vi "Module - Page Login.vi"(11 "Stop":bool) -> ()   [LabVIEW 2020]
uses:
  Control/State - eFGV.ctl
  visinergy_PRSB1-vsys-platform-6e171cc53fe6/VI/HMI/Control/State - Page Login.ctl
  <vilib>/addons/database/NI_Database_API.lvlib
  <vilib>/addons/database/Connection.llb/Conn ObjectReference.ctl
  <vilib>/addons/database/Connection.llb/DB Tools Open Connec (String).vi
  Control/Active Dir Info.ctl
panel:
  out "DB Connected":bool=TRUE
  in  "String.StationID":string
  in  "Button.Stop":bool
  in  "RSS Operation":T1(ring)
  in  "Button.Login":bool
  in  "ComboBox.Domain":string(combo) caption="Domain"
  in  "String.Password":string caption="Password"
  in  "String.Username":string caption="Username"
  in  "String.StationDescription":string
  in  "ComboBox.Station":string(combo) caption="Station"
  in  "String.PlantDescription":string
  in  "ComboBox.Plant":string(combo) caption="Plant"
  in  "Button.ConnectDB":bool
  out "2D data":string[][](array[string])
  in  "DB Connection Info":T2={"Connection"="SRTRS", "Username"="srtrsoss", "Password"="12345"}
  out "standard output":string
  out "Logon OK":bool
  out "Active Dir. Info":T3
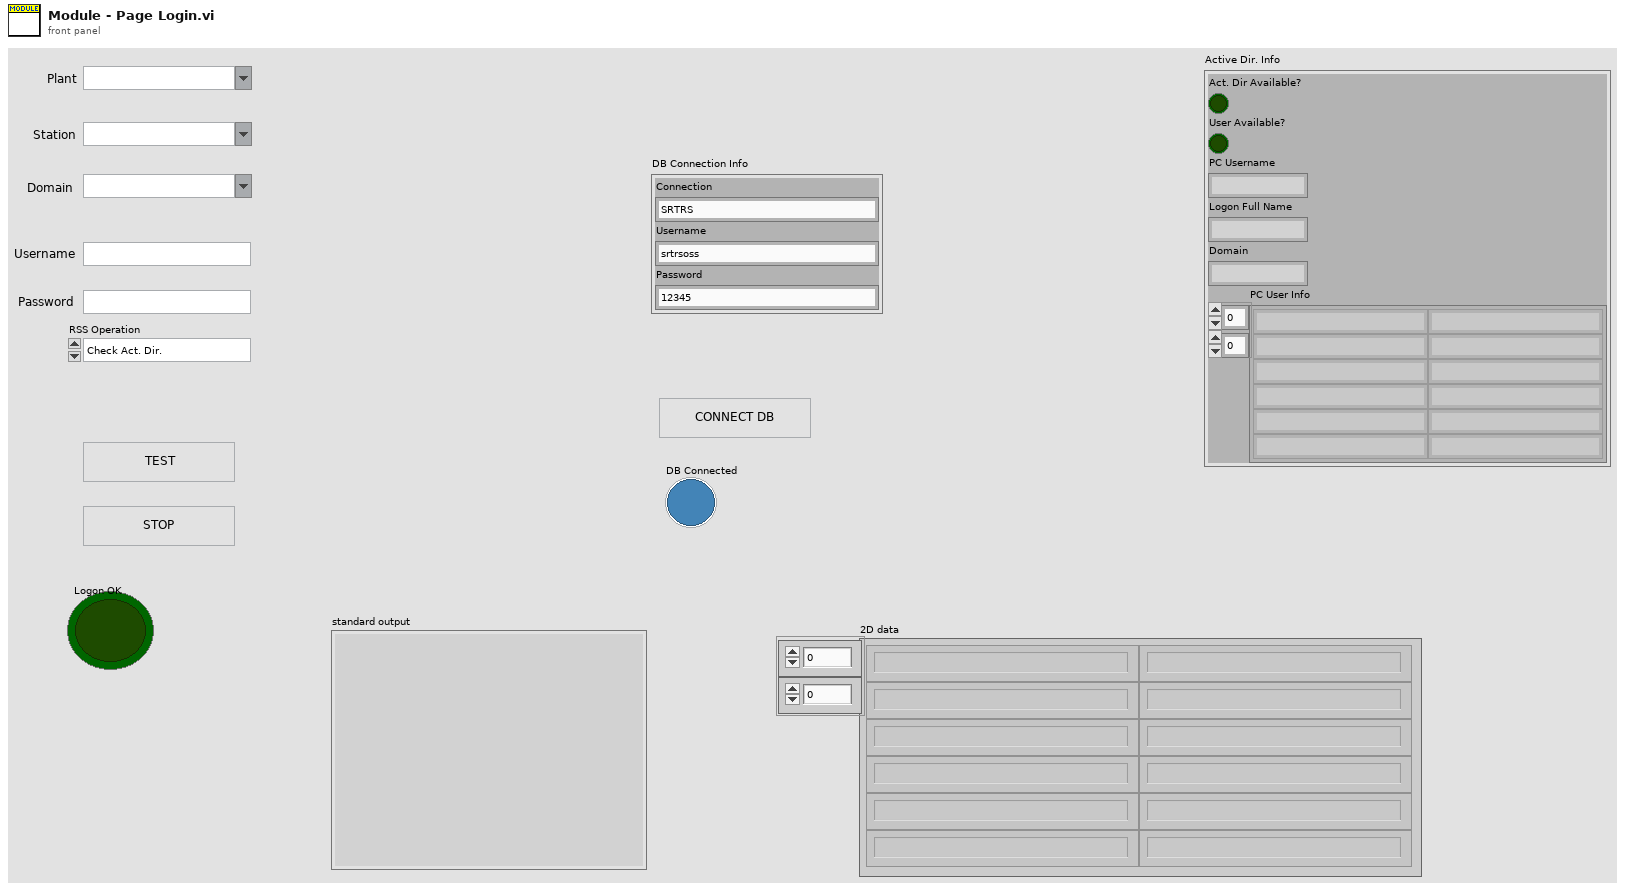
[diagram p1: front panel]
types:
  T1 = enum16{"Check Act. Dir.", "Logon", "PC User", "PC User Info", "Hostname"}
  T2 = cluster{"Connection":string, "Username":string, "Password":string}
  T3 = typedef "Active Dir Info.ctl" = cluster{"Act. Dir Available?":bool, "User Available?":bool, "PC Username":string, "Logon Full Name":string, "Domain":string, "PC User Info":string[][]}
  T4 = typedef "NI_Database_API.lvlib/Conn ObjectReference.ctl" = refnum<k1>
  T5 = cluster{"T_Out":i32, "Event Ref":refnum<event-registration>, "DB Connection Ref":T4, "2D data":string[][]}
  T6 = typedef "State - Page Login.ctl" = enum16{"Init", "Register Event", "Open DB Ref", "Get Info - Plant And Station", "Get Info - Domain", "Idle", "Login", "Close"}
  T7 = typedef "State - eFGV.ctl" = enum16{"Init", "Read", "Write", "Exit"}
  T8 = typedef "eventvkey.ctl" = enum16{"ASCII", "Enter", "Return", "Shift", "Ctrl", "Alt", "Cmd", "Opt", "Caps", "NumLock", "Clear", "Break", "Up", "Down", "Left", "Right", "Insert", "Delete", "Home", "End", "PageUp", "PageDown", "Escape", "Help", "Pause", "ScrollLock", "F1", "F2", "F3", "F4", "F5", "F6", "F7", "F8", "F9", "F10", "F11", "F12", "F13", "F14", "F15", "F16", "F17", "F18", "F19", "F20", "F21", "F22", "F23", "F24", "Play", "VolumeUp", "VolumeDown", "Mute", "Two Byte Char"}
  T9 = enum32{"invalid app kind", "Development System", "Run Time System", "Student Edition", "Embedded LabVIEW", "Evaluation", "Custom"}
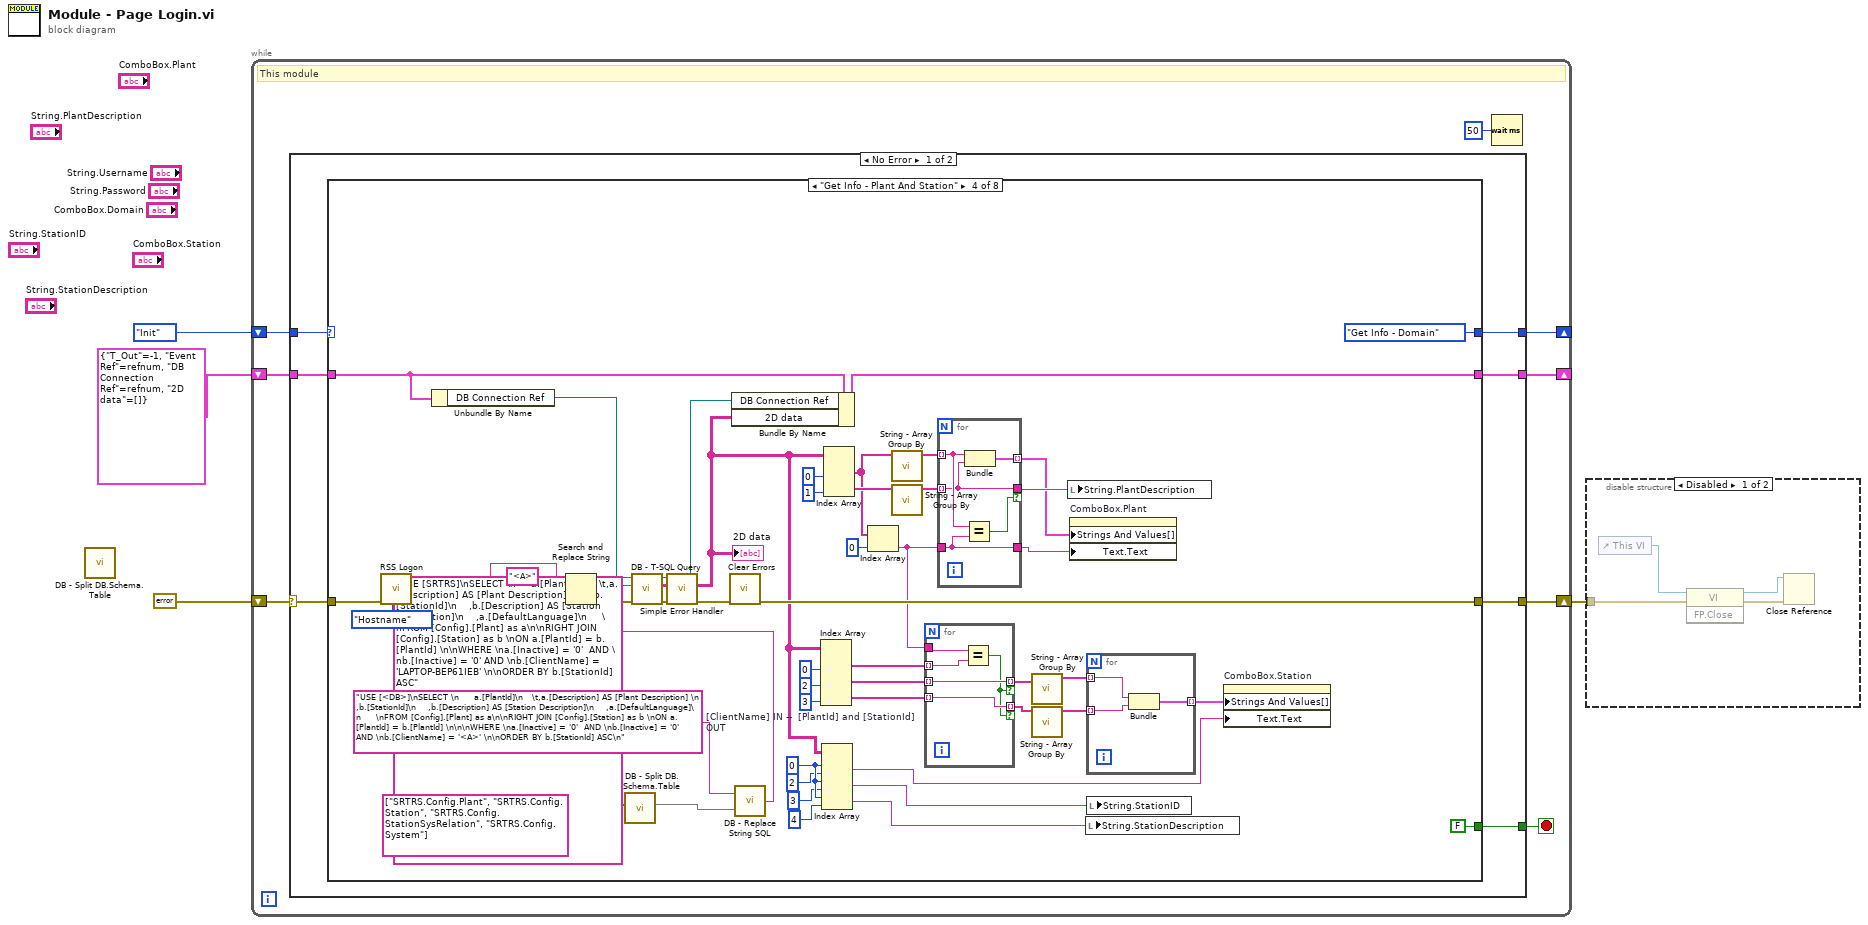
[diagram p0: block diagram]
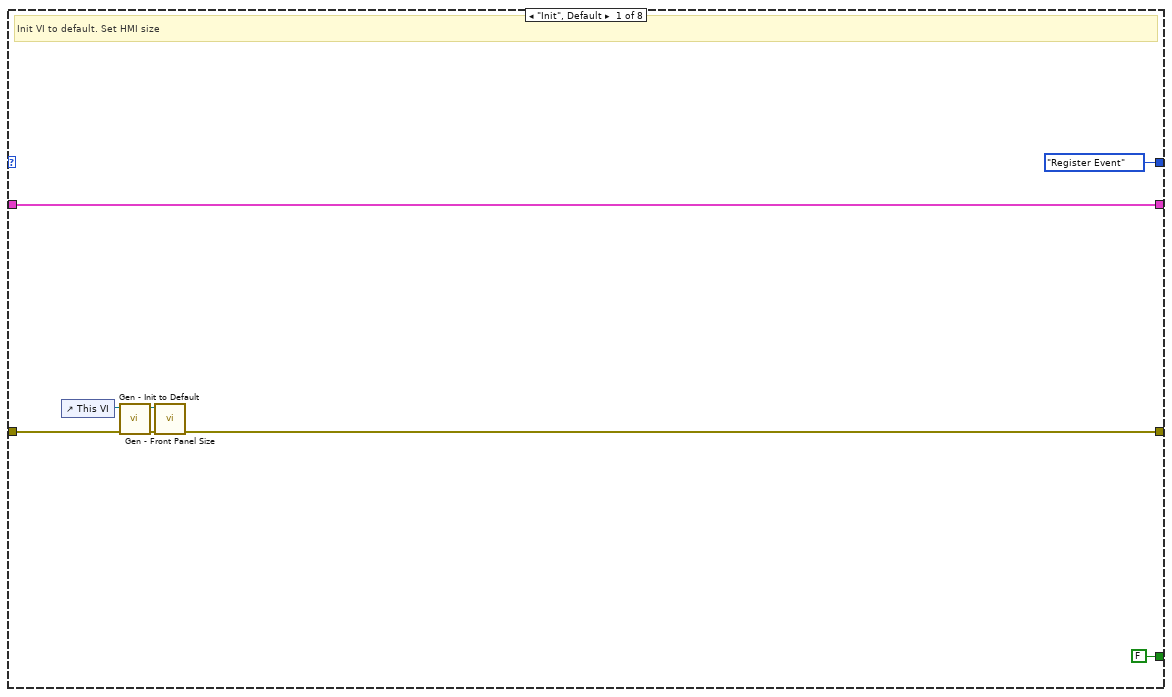
[diagram p3: hidden frame]
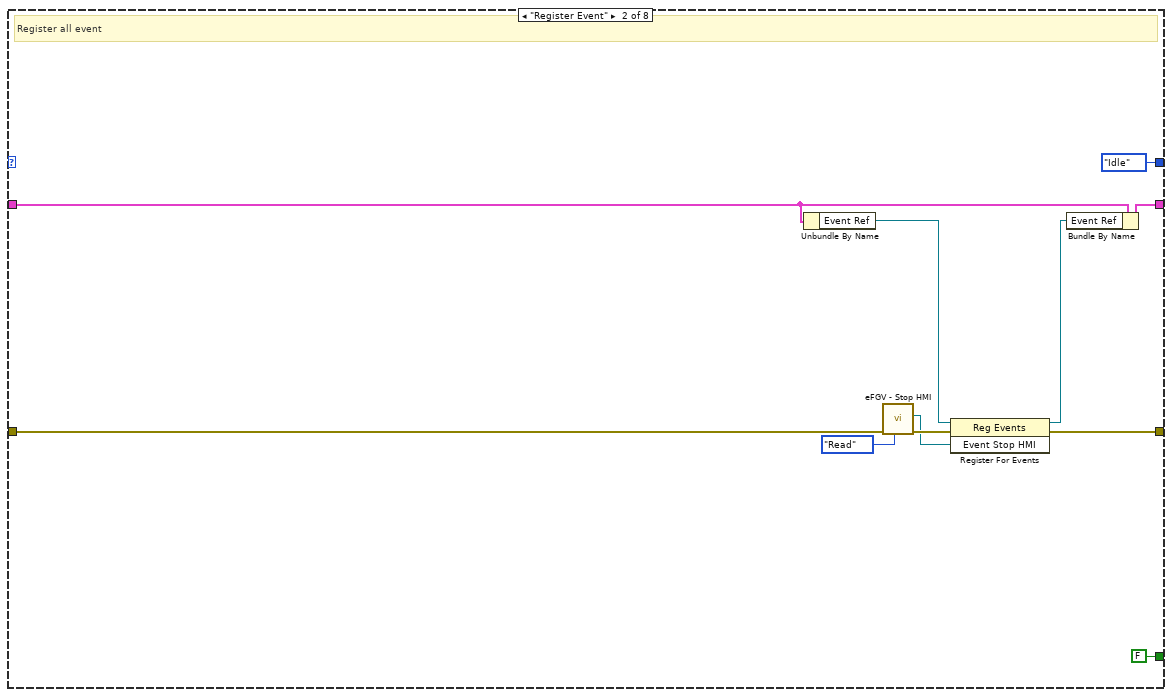
[diagram p4: hidden frame]
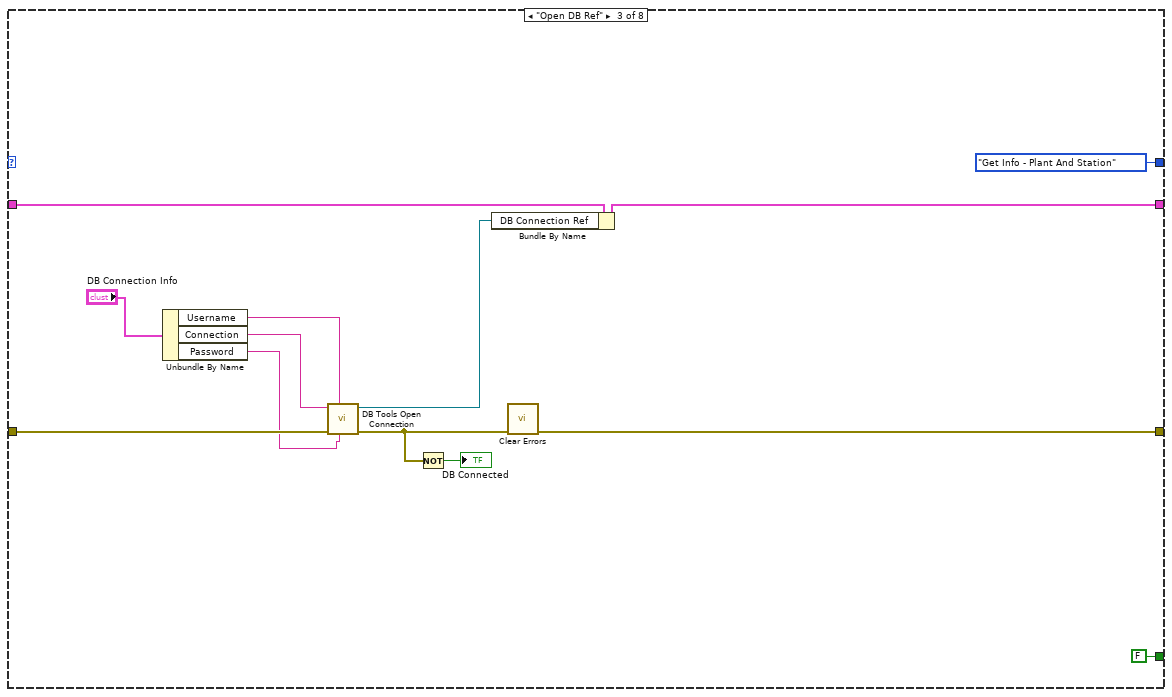
[diagram p5: hidden frame]
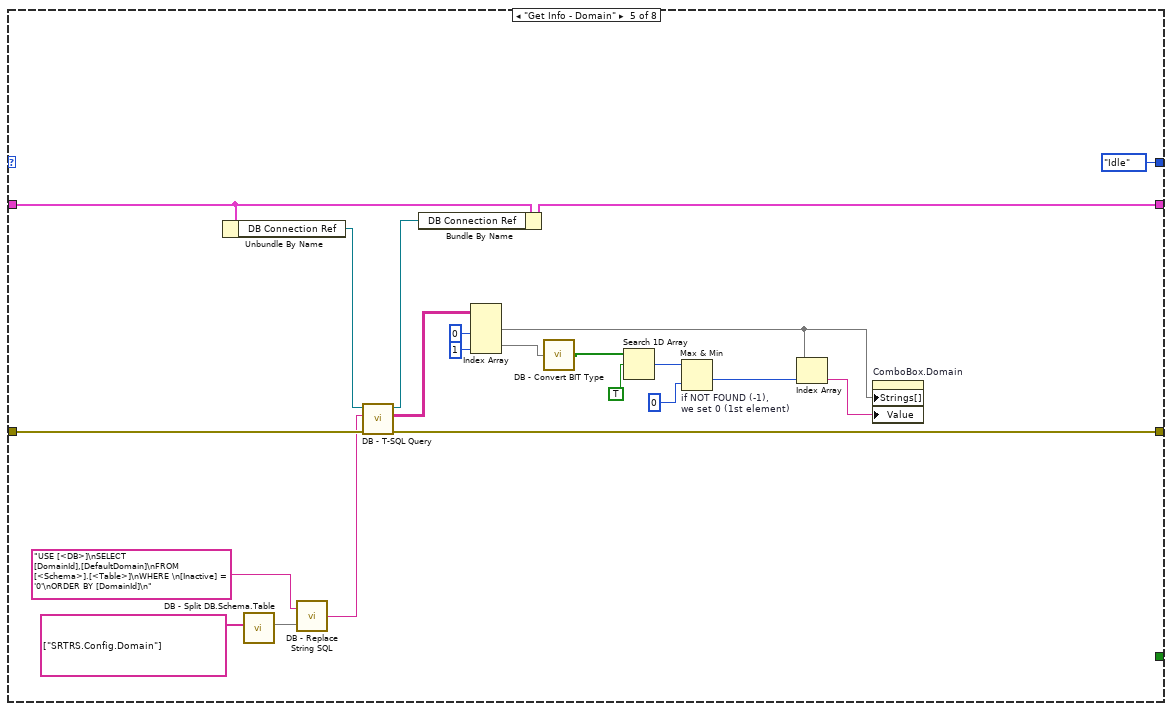
[diagram p6: hidden frame]
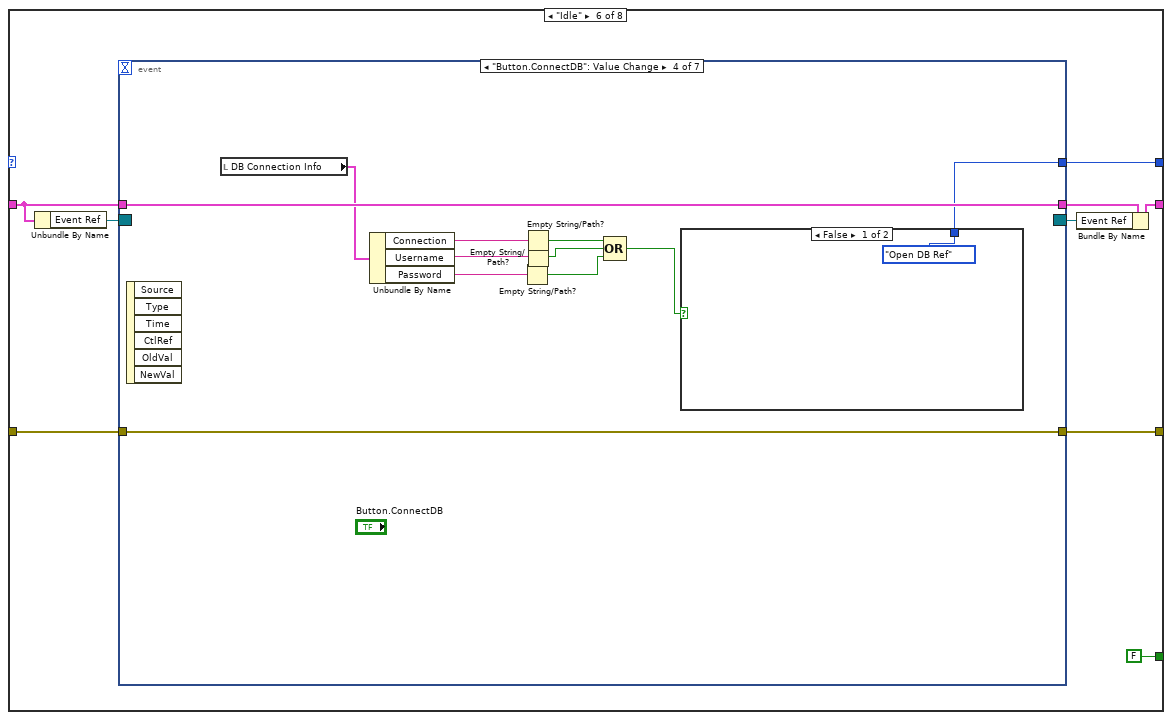
[diagram p7: hidden frame]
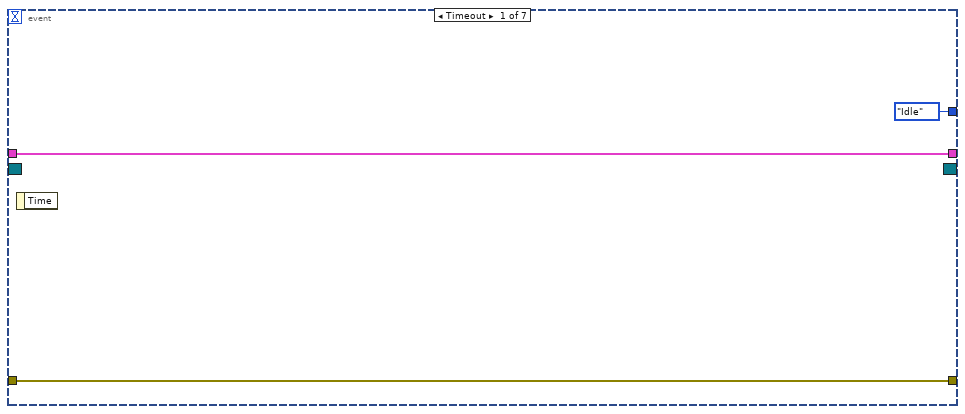
[diagram p8: hidden frame]
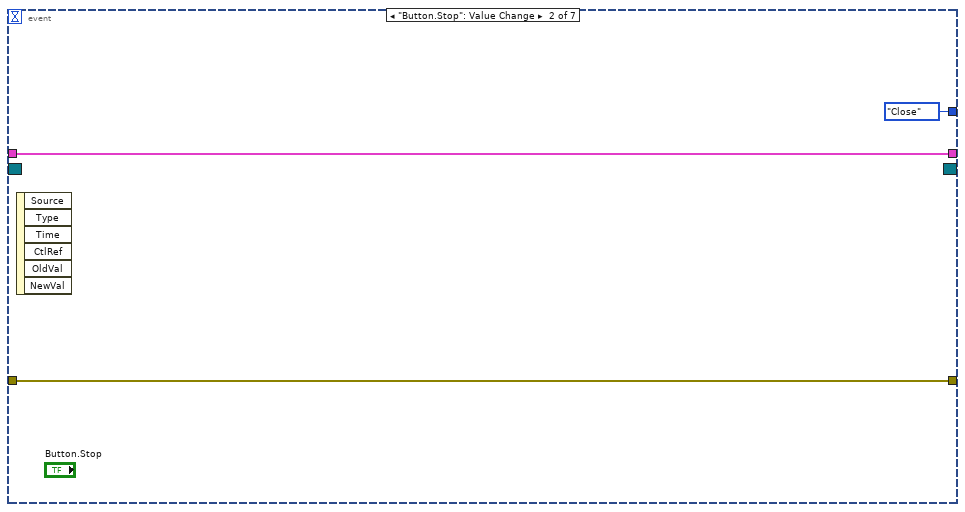
[diagram p9: hidden frame]
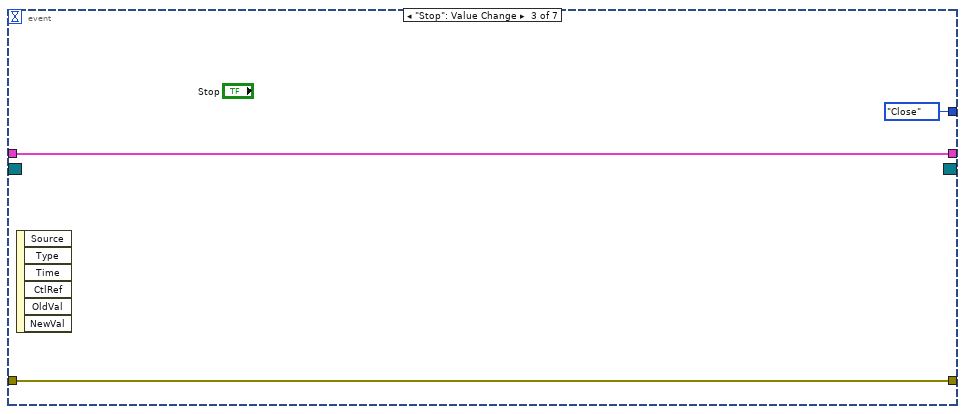
[diagram p10: hidden frame]
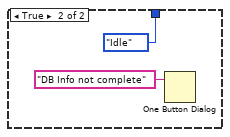
[diagram p11: hidden frame]
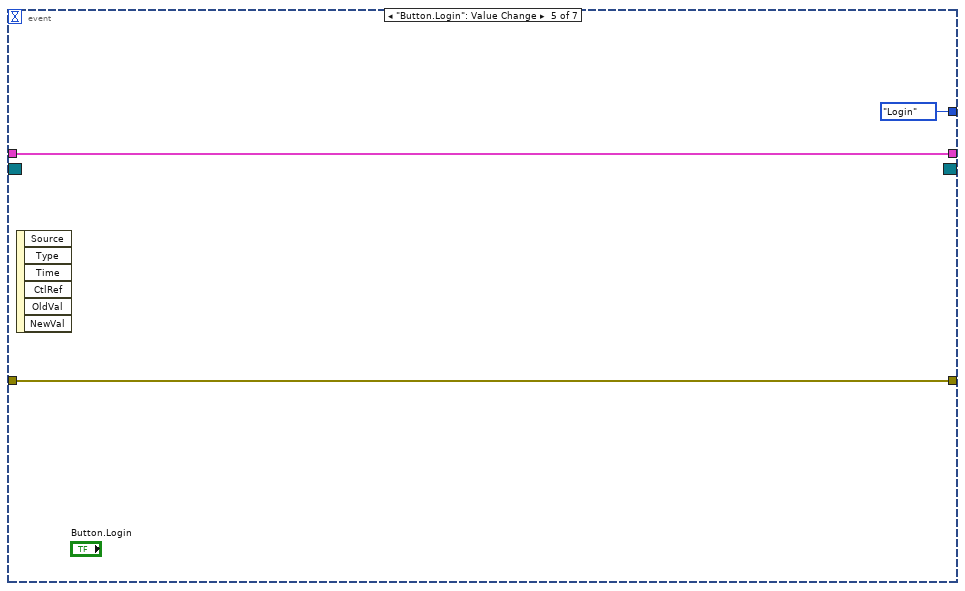
[diagram p12: hidden frame]
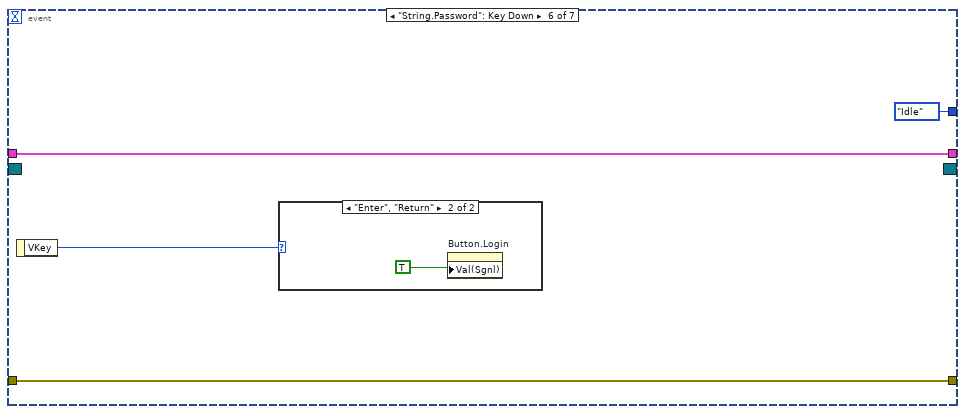
[diagram p13: hidden frame]
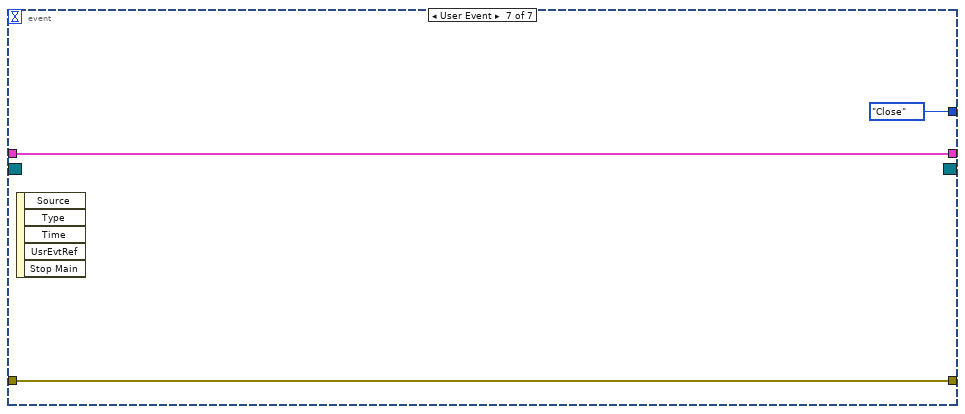
[diagram p15: hidden frame]
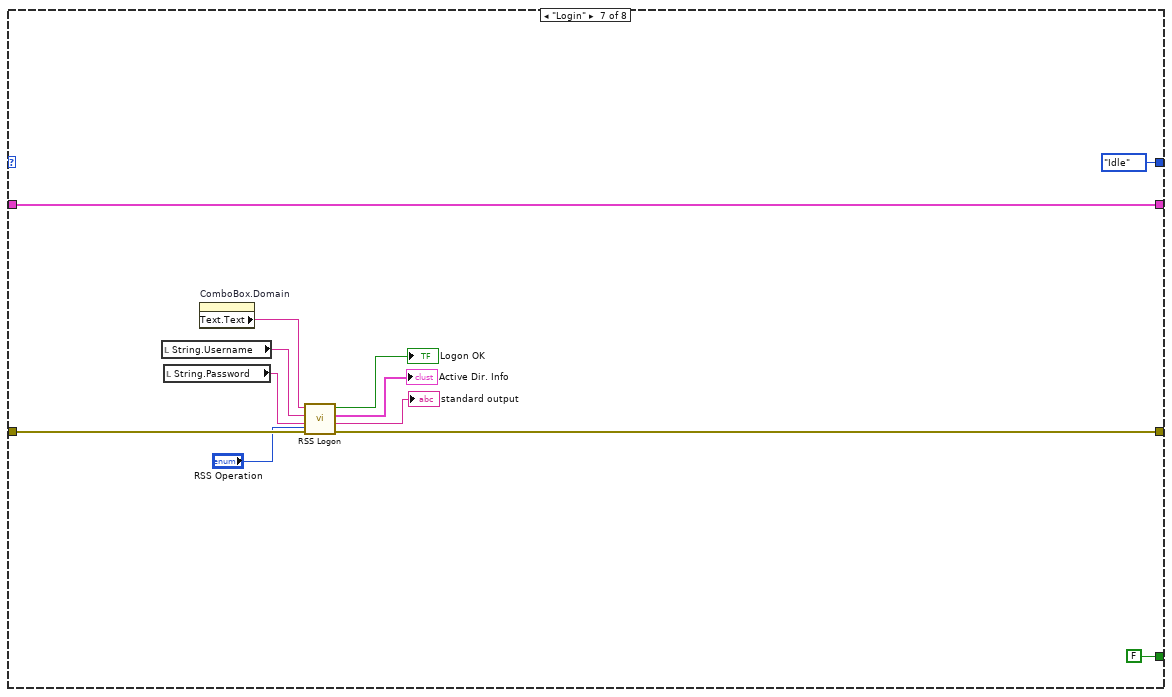
[diagram p16: hidden frame]
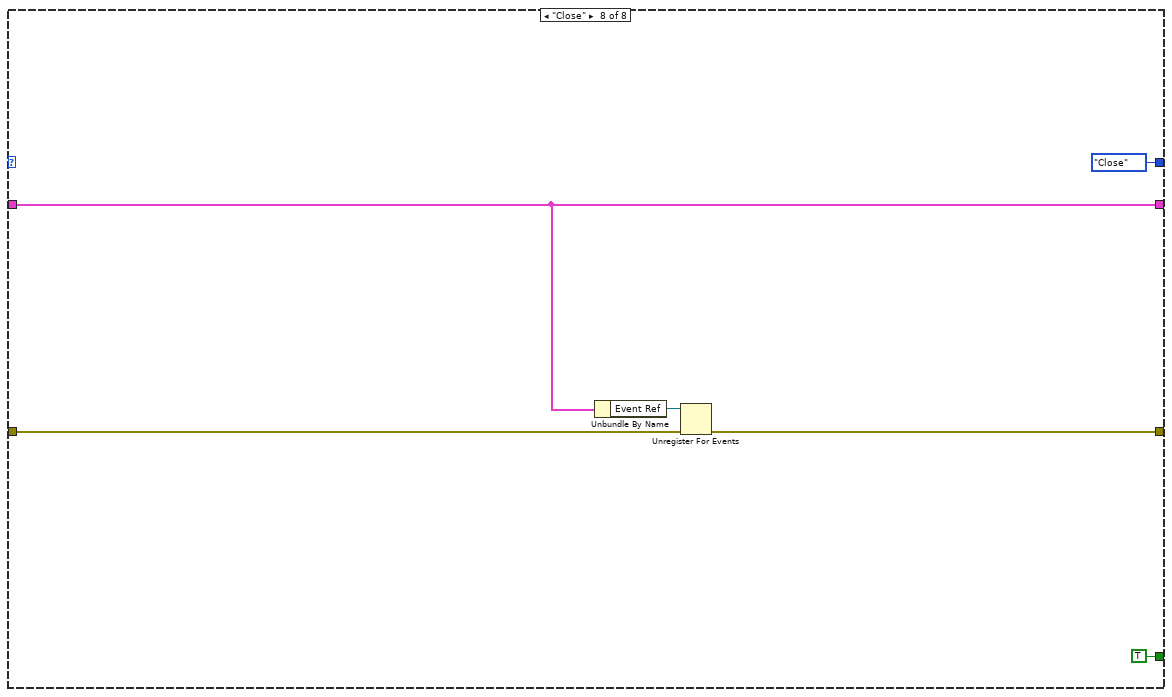
[diagram p17: hidden frame]
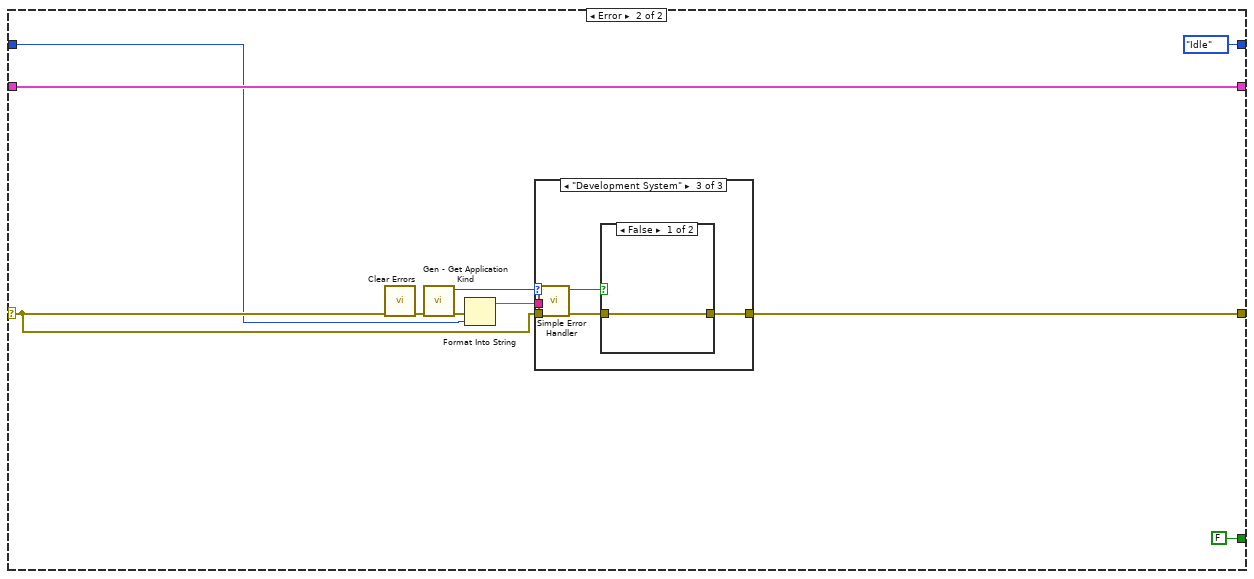
[diagram p18: hidden frame]
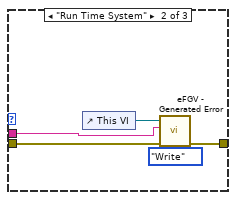
[diagram p20: hidden frame]
diagram:
  n1 = call "DB - Split DB.Schema.Table.vi"() -> ()  [unwired: 11 in, 1 out]
  n2 = while {
    shift-right: [w11] -> w2
    shift-left: errorcluster {"status"=FALSE, "code"=0, "source"=""} ("Error In") -> [w12]
    shift-right: [w8] -> _
    shift-left: T5 {"T_Out"=-1, "Event Ref"=refnum, "DB Connection Ref"=refnum, "2D data"=[]} -> [w9]
    shift-right: [w5] -> _
    shift-left: State_-_Page_Login."Init" -> [w6]
    stop <- w10 stop-if-true
    # "This module"
    n3 = case shown="No Error" w12 {
      selector: w12 -> [w18 w202]
      tunnel: [w19 w203] -> w11
      tunnel: [w17 FALSE] -> w10
      tunnel: w9 -> [w16 w206]
      tunnel: [w15 w206] -> w8
      tunnel: w6 -> [w14 w198]
      tunnel: [w13 State_-_Page_Login."Idle"] -> w5
      frame No Error {
        n4 = case shown="\"Get Info - Plant And Station\"" w14 {
          tunnel: [w25 w38 w41 w84 w132 w145 w188 w196] -> w19
          tunnel: w18 -> [w27 w36 w49 w98 w133 w144 w189 w197]
          tunnel: [FALSE FALSE FALSE FALSE _ FALSE FALSE TRUE] -> w17
          tunnel: w16 -> [w24 w32 w51 w90 w130 w141 w190 w194]
          tunnel: [w24 w30 w48 w86 w128 w139 w190 w194] -> w15
          tunnel: [State_-_Page_Login."Register Event" State_-_Page_Login."Idle" State_-_Page_Login."Get Info - Plant And Station" State_-_Page_Login."Get Info - Domain" State_-_Page_Login."Idle" w137 State_-_Page_Login."Idle" State_-_Page_Login."Close"] -> w13
          frame "Init", Default {
            # "Init VI to default. Set HMI size"
            n5 = control-ref of="This VI"() -> (w22:refnum<vi>)
            n6 = call "Gen - Init to Default.vi"("Error in"=w27, "This VI"=w22) -> ("Error out"=w26:errorcluster, "This VI Copy"=w21:refnum<vi>)  [unwired: 8 in]
            n7 = call "Gen - Front Panel Size.vi"("Error In"=w26, "This VI"=w21) -> ("Error Out"=w25:errorcluster)  [unwired: 9 in]
          }
          frame "Register Event" {
            # "Register all event"
            n8 = Unbundle By Name(w32) -> ("Event Ref"=w31:refnum<event-registration>)
            n9 = call "eFGV - Stop HMI.vi"("Action"=State_-_eFGV."Read", "Error In"=w36) -> ("Error Out"=w37:errorcluster, "Event Stop HMI"=w34:refnum<user-event>)  [unwired: 7 in, 1 out]
            n10 = register-events(reference=w31, error in=w37, w34) -> (reference out=w29:refnum<event-registration>, error out=w38:errorcluster)
            n11 = Bundle By Name(cluster=w32, "Event Ref"=w29) -> (w30:T5)
          }
          frame "Open DB Ref" {
            n12 = Unbundle By Name("DB Connection Info") -> ("Username"=w44:string, "Connection"=w45:string, "Password"=w43:string)
            n13 = call-poly <vilib>:"DB Tools Open Connection.vi"("password"=w43, "userID"=w44, "error in (no error)"=w49, "connection information"=w45) -> ("error out"=w40:errorcluster, "connection reference"=w47:T4)  [unwired: 4 in]
            n14 = Not(x=w40) -> (.not. x?=→"DB Connected":bool)
            n15 = Bundle By Name(cluster=w51, "DB Connection Ref"=w47) -> (w48:T5)
            n16 = call <vilib>:"Clear Errors.vi"("error in (no error)"=w40) -> ("error out"=w41:errorcluster)  [unwired: 5 in, 1 out]
          }
          frame "Get Info - Plant And Station" {
            w60 = 0 ("index (row)")
            w99 = "USE [<DB>]\nSELECT \n     a.[PlantId]\n   \t,a.[Description] AS [Plant Description] \n    ,b.[StationId]\n    ,b.[Description] AS [Station Description]\n    ,a.[DefaultLanguage]\n     \nFROM [Config].[Plant] as a\n\nRIGHT JOIN [Config].[Station] as b \nON a.[PlantId] = b.[PlantId] \n\n\nWHERE \na.[Inactive] = '0'  AND \nb.[Inactive] = '0' AND \nb.[ClientName] = '<A>' \n\nORDER BY b.[StationId] ASC\n"  # [ClientName] IN --  [PlantId] and [StationId] OUT
            n17 = call "RSS Logon.vi"("RSS Operation"=T1."Hostname", "error in (no error)"=w98) -> ("error out"=w96:errorcluster, "standard output"=w93:string)  [unwired: 6 in, 2 out]
            n18 = Unbundle By Name(w90) -> ("DB Connection Ref"=w87:T4)
            n19 = call "DB - Split DB.Schema.Table.vi"(10:string[] ["SRTRS.Config.Plant", "SRTRS.Config.Station", "SRTRS.Config.StationSysRelation", "SRTRS.Config.System"] ("DB.Schema.Table String")) -> (2:w100)  [unwired: 9 in, 1 out]
            n20 = call "DB - Replace String SQL.vi"("DB.Schema.Table"=w100, "String In"=w99) -> ("String Out"=w95:string)
            n21 = Search and Replace String(input string=w95, search string="<A>", replace string=w93, error in=w96) -> (error out=w89:errorcluster)  [unwired: 4 in, 3 out]
            n22 = call "DB - T-SQL Query.vi"("error in (no error)"=w89, "T-SQL"="USE [SRTRS]\nSELECT \n     a.[PlantId]\n   \t,a.[Description] AS [Plant Description] \n    ,b.[StationId]\n    ,b.[Description] AS [Station Description]\n    ,a.[DefaultLanguage]\n     \nFROM [Config].[Plant] as a\n\nRIGHT JOIN [Config].[Station] as b \nON a.[PlantId] = b.[PlantId] \n\nWHERE \na.[Inactive] = '0'  AND \nb.[Inactive] = '0' AND \nb.[ClientName] = 'LAPTOP-BEP61IEB' \n\nORDER BY b.[StationId] ASC", "connection reference"=w87) -> ("error out"=w88:errorcluster, "2D data"=w61:string[][], "connection reference"=w85:T4)  [unwired: 6 in]
            "2D data" <- w61
            n23 = call <vilib>:"Simple Error Handler.vi"("error in (no error)"=w88) -> ("error out"=w53:errorcluster)  [unwired: 4 in, 4 out]
            n24 = call <vilib>:"Clear Errors.vi"("error in (no error)"=w53) -> ("error out"=w84:errorcluster)  [unwired: 5 in, 1 out]
            n25 = Bundle By Name(cluster=w90, "DB Connection Ref"=w85, "2D data"=w61) -> (w86:T5)
            n26 = Index Array(array=w61, index (col) #1=0 ("disabled index (col)"), index (col) #2=2 ("index (col)"), index (col) #3=3 ("index (col)")) -> (element #1=w70:string[], element #2=w69:string[], element #3=w68:string[])  [unwired: 3 in]
            n27 = Index Array(array=w61, index (row) #1=w60, index (col) #1=2 ("disabled index (col)"), index (row) #2=w60, index (col) #2=3 ("disabled index (col)"), index (row) #3=w60, index (col) #3=4 ("disabled index (col)")) -> (element #1=w56:string, element #2=w55:string, element #3=w54:string)
            n28 = Index Array(array=w61, index (col) #1=0 ("disabled index (col)"), index (col) #2=1 ("index (col)")) -> (element #1=w78:string[], element #2=w81:string[])  [unwired: 2 in]
            n29 = Index Array(array=w78, index=0) -> (element=w67:string)
            n30 = call "String - Array Group By.vi"("Array in"=w78) -> ("GROUP BY (Array in)"=w80:string[])  [unwired: 10 in]
            n31 = call "String - Array Group By.vi"("Array in"=w81) -> ("GROUP BY (Array in)"=w79:string[])  [unwired: 10 in]
            n32 = for {
              tunnel: w70 -> [w108] mode=indexing
              tunnel: w69 -> [w107] mode=indexing
              tunnel: w68 -> [w106] mode=indexing
              tunnel: w67 -> [w109]
              tunnel: [w107] -> w66 mode=indexing if=w105
              tunnel: [w106] -> w65 mode=indexing if=w105
              n33 = Equal?(x=w109, y=w108) -> (x = y?=w105:bool)
            }
            n34 = for {
              tunnel: w80 -> [w113] mode=indexing
              tunnel: w79 -> [w112] mode=indexing
              tunnel: [w114] -> w75 mode=indexing
              tunnel: w67 -> [w110]
              tunnel: [w112] -> w76 if=w111
              tunnel: [w110] -> w74
              n35 = Equal?(x=w113, y=w110) -> (x = y?=w111:bool)
              n36 = Bundle("String"=w113, "String"=w112) -> (w114:cluster{"String":string, "String":string})  [unwired: 1 in]
            }
            n37 = call "String - Array Group By.vi"("Array in"=w66) -> ("GROUP BY (Array in)"=w64:string[])  [unwired: 10 in]
            n38 = call "String - Array Group By.vi"("Array in"=w65) -> ("GROUP BY (Array in)"=w63:string[])  [unwired: 10 in]
            n39 = local write "String.PlantDescription"(w76) -> ()
            n40 = property on="ComboBox.Plant" class="CmbBox"("Strings And Values[]"=w75, "Text.Text"=w74) -> ()  [unwired: 2 in, 2 out]
            n41 = local write "String.StationDescription"(w54) -> ()
            n42 = for {
              tunnel: w64 -> [w104] mode=indexing
              tunnel: w63 -> [w103] mode=indexing
              tunnel: [w102] -> w62 mode=indexing
              n43 = Bundle("String"=w104, "String"=w103) -> (w102:cluster{"String":string, "String":string})  [unwired: 1 in]
            }
            n44 = local write "String.StationID"(w55) -> ()
            n45 = property on="ComboBox.Station" class="CmbBox"("Strings And Values[]"=w62, "Text.Text"=w56) -> ()  [unwired: 2 in, 2 out]
          }
          frame "Get Info - Domain" {
            n46 = Unbundle By Name(w130) -> ("DB Connection Ref"=w129:T4)
            n47 = call "DB - Split DB.Schema.Table.vi"(10:string[] ["SRTRS.Config.Domain"] ("DB.Schema.Table String")) -> (2:w135)  [unwired: 9 in, 1 out]
            n48 = call "DB - Replace String SQL.vi"("DB.Schema.Table"=w135, "String In"="USE [<DB>]\nSELECT [DomainId],[DefaultDomain]\nFROM [<Schema>].[<Table>]\nWHERE \n[Inactive] = '0'\nORDER BY [DomainId]\n") -> ("String Out"=w131:string)
            n49 = call "DB - T-SQL Query.vi"("error in (no error)"=w133, "T-SQL"=w131, "connection reference"=w129) -> ("error out"=w132:errorcluster, "2D data"=w126:string[][], "connection reference"=w127:T4)  [unwired: 6 in]
            n50 = Bundle By Name(cluster=w130, "DB Connection Ref"=w127) -> (w128:T5)
            n51 = Index Array(array=w126, index (col) #1=0 ("disabled index (col)"), index (col) #2=1 ("index (col)")) -> (element #1=w117:string[], element #2=w123:string[])  [unwired: 2 in]
            n52 = call "DB - Convert BIT Type.vi"("BIT Type (eg Inactive) (Array)"=w123) -> ("Boolean (Array)"=w118:bool[])  [unwired: 2 in, 2 out]
            n53 = Search 1D Array(1D array=w118, element=TRUE) -> (index of element=w120:i32)  [unwired: 1 in]
            n54 = Max & Min "if NOT FOUND (-1),\nwe set 0 (1st element)"(x=w120, y=0) -> (max(x,y)=w121:i32)  [unwired: 1 out]
            n55 = Index Array(array=w117, index=w121) -> (element=w116:string)
            n56 = property on="ComboBox.Domain" class="CmbBox"("Strings[]"=w117, "Value"=w116) -> ()  [unwired: 2 in, 2 out]
          }
          frame "Idle" {
            n57 = Unbundle By Name(w141) -> ("Event Ref"=w140:refnum<event-registration>)
            n58 = event shown="[3] \"Button.ConnectDB\": Value Change" {
              selector: w140 -> [_ _ _ _ _ _ _]
              dyn-events: [_ _ _ _ _ _ _] -> w138
              timeout: _ -> [_ _ _ _ _ _ _]
              tunnel: [w148 w151 w154 w165 w171 w175 w179] -> w145
              tunnel: w144 -> [w148 w151 w154 w165 w171 w175 w179]
              tunnel: [w147 w150 w153 w164 w170 w174 w178] -> w142
              tunnel: w141 -> [w147 w150 w153 w164 w170 w174 w178]
              tunnel: [State_-_Page_Login."Idle" State_-_Page_Login."Close" State_-_Page_Login."Close" w155 State_-_Page_Login."Login" State_-_Page_Login."Idle" State_-_Page_Login."Close"] -> w137
              event Timeout {
                n59 = event-data() -> ()  [unwired: 1 in, 1 out]
              }
              event "Button.Stop": Value Change {
                n60 = event-data() -> ()  [unwired: 1 in, 6 out]
              }
              event "Stop": Value Change {
                n61 = event-data() -> ()  [unwired: 1 in, 6 out]
              }
              event "Button.ConnectDB": Value Change {
                n62 = event-data() -> ()  [unwired: 1 in, 6 out]
                n63 = local read "DB Connection Info"() -> (w163:T2)
                n64 = Unbundle By Name(w163) -> ("Connection"=w162:string, "Username"=w161:string, "Password"=w160:string)
                n65 = Empty String/Path?(string/path=w160) -> (empty?=w157:bool)
                n66 = Empty String/Path?(string/path=w162) -> (empty?=w159:bool)
                n67 = Empty String/Path?(string/path=w161) -> (empty?=w158:bool)
                n68 = Compound Arithmetic op=OR(w159, w158, w157) -> (w156:bool)
                n69 = case shown="False" w156 {
                  tunnel: [State_-_Page_Login."Open DB Ref" State_-_Page_Login."Idle"] -> w155
                  frame False {
                  }
                  frame True {
                    n70 = One Button Dialog(message="DB Info not complete") -> ()  [unwired: 1 in, 1 out]
                  }
                }
              }
              event "Button.Login": Value Change {
                n71 = event-data() -> ()  [unwired: 1 in, 6 out]
              }
              event "String.Password": Key Down {
                n72 = event-data() -> ("VKey"=w173:T8)  [unwired: 1 in]
                n73 = case shown="\"Enter\", \"Return\"" w173 {
                  frame "ASCII", Default {
                  }
                  frame "Enter", "Return" {
                    n74 = property on="Button.Login" class="Bool"("Val(Sgnl)"=TRUE) -> ()  [unwired: 2 in, 2 out]
                  }
                }
              }
              event User Event {
                n75 = event-data() -> ()  [unwired: 1 in, 5 out]
              }
            }
            n76 = Bundle By Name(cluster=w142, "Event Ref"=w138) -> (w139:T5)
          }
          frame "Login" {
            n77 = local read "String.Username"() -> (w183:string)
            n78 = local read "String.Password"() -> (w182:string)
            n79 = property on="ComboBox.Domain" class="CmbBox"() -> ("Text.Text"=w180:string)  [unwired: 2 in, 2 out]
            n80 = call "RSS Logon.vi"("RSS Operation"="RSS Operation", "error in (no error)"=w189, "Password"=w182, "Logon User"=w183, "Domain"=w180) -> ("error out"=w188:errorcluster, "standard output"=→"standard output":string, "Active Dir. Info"=→"Active Dir. Info":T3, "Logon OK"=→"Logon OK":bool)  [unwired: 3 in]
          }
          frame "Close" {
            n81 = Unbundle By Name(w194) -> ("Event Ref"=w193:refnum<event-registration>)
            n82 = Unregister For Events(event registration refnum=w193, error in=w197) -> (error out=w196:errorcluster)
          }
        }
      }
      frame Error {
        n83 = call <vilib>:"Clear Errors.vi"("error in (no error)"=w202) -> ("error out"=w205:errorcluster)  [unwired: 5 in, 1 out]
        n84 = call "Gen - Get Application Kind.vi"("Error In"=w205) -> ("Error Out"=w201:errorcluster, "Application:Kind"=w204:T9)  [unwired: 9 in]
        n85 = Format Into String(error in=w201, w198) -> (resulting string=w200:string)  [unwired: 2 in, 1 out]
        n86 = case shown="\"Development System\"" w204 {
          tunnel: [w208 w213 w217] -> w203
          tunnel: w202 -> [w208 w210 w215]
          tunnel: w200 -> [_ w209 _]
          frame "invalid app kind", Default {
          }
          frame "Run Time System" {
            n87 = control-ref of="This VI"() -> (w211:refnum<vi>)
            n88 = call "eFGV - Generated Error.vi"("eFGV States"=State_-_eFGV."Write", "Error In"=w210, "State"=w209, "This VI"=w211) -> ("Error Out"=w213:errorcluster)  [unwired: 6 in, 1 out]
          }
          frame "Development System" {
            n89 = call <vilib>:"Simple Error Handler.vi"("error in (no error)"=w215) -> ("error?"=w214:bool, "error out"=w216:errorcluster)  [unwired: 4 in, 3 out]
            n90 = case shown="False" w214 {
              tunnel: [w218 w220] -> w217
              tunnel: w216 -> [w218 w219]
              frame False {
              }
              frame True {
                n91 = call <vilib>:"Clear Errors.vi"("error in (no error)"=w219) -> ("error out"=w220:errorcluster)  [unwired: 5 in, 1 out]
              }
            }
          }
        }
      }
    }
    n92 = Wait (ms)(milliseconds to wait=u32 50) -> ()  [unwired: 1 out]
  }
  n93 = disable-structure shown="Disabled" {
    disable-tunnel: w2 -> [w224 _]
    frame Disabled {
      n94 = control-ref of="This VI"() -> (w223:refnum<vi>)
      n95 = invoke class="VI" method="FP.Close"(reference=w223, error in=w224) -> (reference out=w221:refnum<vi>, error out=w222:errorcluster)  [unwired: 1 in, 1 out]
      n96 = Close Reference(reference=w221, error in (no error)=w222) -> ()  [unwired: 1 out]
    }
    frame Enabled {
    }
  }
